vi "Test HELP API.vi"() -> ()   [LabVIEW 2019, in "Inst.Transport.lvclass"]
uses:
  Inst.Transport.lvclass
  C:/Program Files (x86)/National Instruments/LabVIEW 2019/user.lib/LevyLab/Instrument Framework/Instrument/Instrument.lvclass
  <userlib>/LevyLab/Instrument Framework/Instrument/Instrument.lvclass
panel:
  out "Array":string[](array[string])
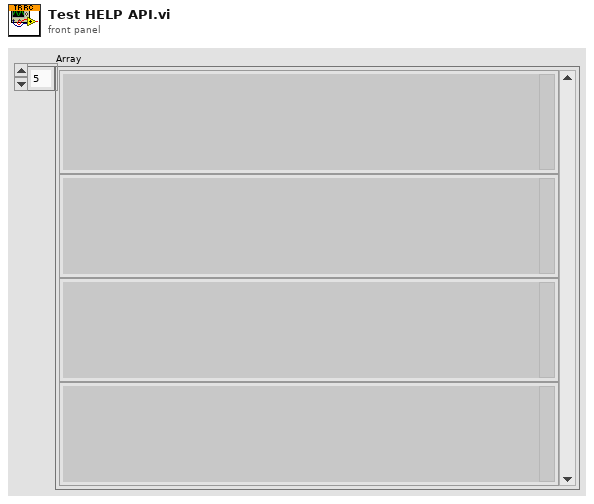
[diagram p1: front panel]
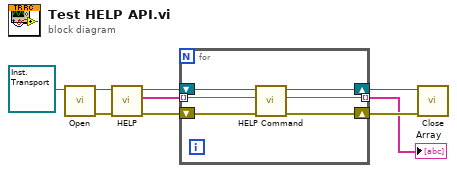
[diagram p0: block diagram]
diagram:
  n1 = call-dynamic "Open.vi"("Inst.Transport in"=refnum<class "Inst.Transport.lvclass"> refnum) -> ("error out"=w9:errorcluster, "Inst.Transport out"=w8:refnum<class "Inst.Transport.lvclass">)  [unwired: 9 in]
  n2 = call <userlib>:"HELP.vi"("error in (no error)"=w9, "Instrument in"=w8) -> ("error out"=w6:errorcluster, "Commands"=w2:string[], "Instrument in"=w5:refnum<class "Inst.Transport.lvclass">)  [unwired: 7 in]
  n3 = for {
    shift-right: [w12] -> w3
    shift-left: w6 -> [w15]
    shift-right: [w13] -> w4
    shift-left: w5 -> [w14]
    tunnel: w2 -> [w11] mode=indexing
    tunnel: [w10] -> w1 mode=indexing
    n4 = call <userlib>:"HELP Command.vi"("error in (no error)"=w15, "command"=w11, "Instrument in"=w14) -> ("error out"=w12:errorcluster, "HELP out"=w10:string, "Instrument in"=w13:refnum<class "Inst.Transport.lvclass">)  [unwired: 6 in]
  }
  "Array" <- w1
  n5 = call-dynamic "Close.vi"("error in (no error)"=w3, "Inst.Transport in"=w4) -> ()  [unwired: 8 in, 2 out]
